vi "test Read Event rtlinux.vi"() -> ()   [LabVIEW 2026]
uses:
  source/PCANBasic.lvlib
  source/Read Event/Read Event.lvclass
  source/PCAN Message types.ctl
  source/PCAN Message.ctl
  source/TPCANHandle.ctl
  source/PCAN Baud.ctl
panel:
  out "Time Stamp":timestamp format="%<%x %.3X>T"
  out "PCAN Message":T1 {"DATA"."7" format="%.0x"; "DATA"."6" format="%.0x"; "DATA"."5" format="%.0x"; "DATA"."4" format="%.0x"; "DATA"."3" format="%.0x"; "DATA"."2" format="%.0x"; "DATA"."1" format="%.0x"; "DATA"."0" format="%.0x"; "MSGTYPE" items=["STANDARD"=0, "RTR"=1, "EXTENDED"=2, "FD"=4, "BRS"=8, "ESI"=16, "ECHO"=32, "ERRFRAME"=64, "STATUS"=128]}
  out "error out":errorcluster
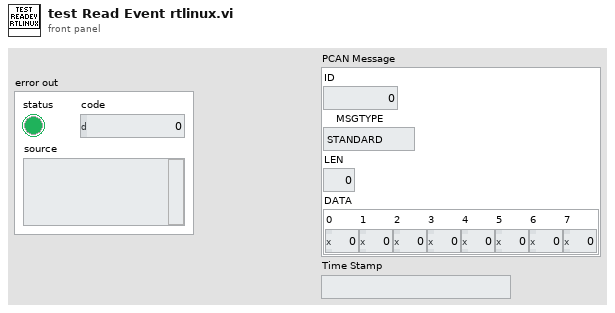
[diagram p1: front panel]
types:
  T1 = typedef "PCANBasic.lvlib/PCAN Message.ctl" = cluster{"ID":u32, "MSGTYPE":T2, "LEN":u8, "DATA":cluster{"0":u8, "1":u8, "2":u8, "3":u8, "4":u8, "5":u8, "6":u8, "7":u8}}
  T2 = typedef "PCANBasic.lvlib/PCAN Message types.ctl" = u8
  T3 = typedef "PCANBasic.lvlib/PCAN Baud.ctl" = u16
  T4 = typedef "PCANBasic.lvlib/TPCANHandle.ctl" = u16
  T5 = cluster{"ID":u32, "MSGTYPE":cluster{"Type":u8, "Extended":bool, "Echo":bool}, "LEN":u8, "DATA":cluster{"0":u8, "1":u8, "2":u8, "3":u8, "4":u8, "5":u8, "6":u8, "7":u8}}
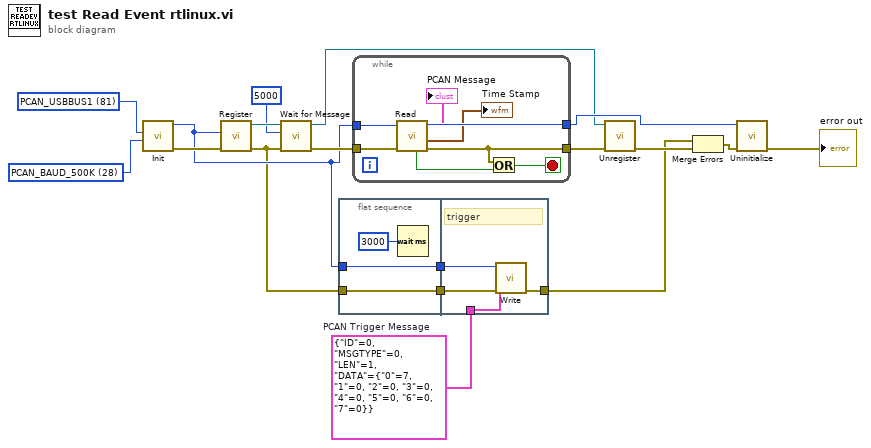
[diagram p0: block diagram]
diagram:
  w2 = T3 28 items=["PCAN_BAUD_1M"=20, "PCAN_BAUD_800K"=22, "PCAN_BAUD_500K"=28, "PCAN_BAUD_250K"=284, "PCAN_BAUD_125K"=796, "PCAN_BAUD_100K"=17199, "PCAN_BAUD_95K"=49998, "PCAN_BAUD_83K"=34091, "PCAN_BAUD_50K"=18223, "PCAN_BAUD_47K"=5140, "PCAN_BAUD_33K"=35631, "PCAN_BAUD_20K"=21295, "PCAN_BAUD_10K"=26415, "PCAN_BAUD_5K"=32639] ("Baudrate")
  w3 = T4 81 items=["PCAN_NONEBUS"=0, "PCAN_USBBUS1"=81, "PCAN_USBBUS2"=82, "PCAN_USBBUS3"=83, "PCAN_USBBUS4"=84, "PCAN_USBBUS5"=85, "PCAN_USBBUS6"=86, "PCAN_USBBUS7"=87, "PCAN_USBBUS8"=88, "PCAN_USBBUS9"=1289, "PCAN_USBBUS10"=1290, "PCAN_USBBUS11"=1291, "PCAN_USBBUS12"=1292, "PCAN_USBBUS13"=1293, "PCAN_USBBUS14"=1294, "PCAN_USBBUS15"=1295, "PCAN_USBBUS16"=1296] ("Channel")
  w9 = T1 {"ID"=0, "MSGTYPE"=0, "LEN"=1, "DATA"={"0"=7, "1"=0, "2"=0, "3"=0, "4"=0, "5"=0, "6"=0, "7"=0}}  # PCAN Trigger Message
  n1 = call "Init.vi"("Baudrate"=w2, "Channel"=w3) -> ("error out"=w16:errorcluster, "TPCANHandle out"=w11:T4)  [unwired: 7 in, 1 out]
  n2 = call "Register.vi"("error in"=w16, "TPCANHandle"=w11) -> ("error out"=w10:errorcluster, "Read Event out"=w15:refnum<class "Read Event.lvclass">)  [unwired: 8 in]
  n3 = call "Wait for Message.vi"("error in"=w10, "Timeout"=u32 5000, "Read Event in"=w15) -> ("error out"=w13:errorcluster, "Read Event out"=w6:refnum<class "Read Event.lvclass">)  [unwired: 6 in, 1 out]
  n4 = flat-sequence {
    tunnel: w11 -> [w20]
    tunnel: [w20] -> w18
    tunnel: w10 -> [w19]
    tunnel: [w19] -> w17
    tunnel: w18 -> [w25]
    tunnel: w17 -> [w24]
    tunnel: [w23] -> w4
    tunnel: w9 -> [w22]
    frame #0 {
      n5 = Wait (ms)(milliseconds to wait=u32 3000) -> ()  [unwired: 1 out]
    }
    frame #1 {
      # "trigger"
      n6 = call "Write.vi"("error in"=w24, "PCAN Message"=w22, "TPCANHandle in"=w25) -> ("error out"=w23:errorcluster)  [unwired: 6 in, 2 out]
    }
  }
  n7 = while {
    tunnel: w11 -> [w33]
    tunnel: w13 -> [w31]
    tunnel: [w26] -> w12
    tunnel: [w30] -> w8
    stop <- w27 stop-if-true
    n8 = call "Read.vi"("error in"=w31, "TPCANHandle in"=w33) -> ("error out"=w26:errorcluster, "Time Stamp"=→"Time Stamp":timestamp, "PCAN Message"=→"PCAN Message":T5, "TPCANHandle out"=w30:T4, "Receive Queue empty"=w32:bool)  [unwired: 4 in, 1 out]
    n9 = Or(x=w26, y=w32) -> (x .or. y?=w27:bool)
  }
  n10 = call "Unregister.vi"("error in"=w12, "Read Event in"=w6) -> ("error out"=w7:errorcluster)  [unwired: 8 in, 1 out]
  n11 = Merge Errors(w4, w7) -> (w5:errorcluster)
  n12 = call "Uninitialize.vi"("error in"=w5, "TPCANHandle in"=w8) -> ("error out"=→"error out":errorcluster)  [unwired: 8 in, 1 out]
